vi "v0.2_vout_serial.vi"(8 "error in (no error)":errorcluster, 10 "Volt":dbl, 11 "VISA COM IN":refnum<visa-resource-name>) -> (0 "error out":errorcluster, 3 "VISA COM OUT":refnum<visa-resource-name>)   [LabVIEW 2011]
doc: "<B>Control de Velocidad</B>\n\nCabia el voltaje a la salida del amplificador operacional. Esto controla la velocidad del servomotor cuando se lo configura en modo de Control de Velocidad\n<B>Vout</B> Un valor entre -10 y 10 V"
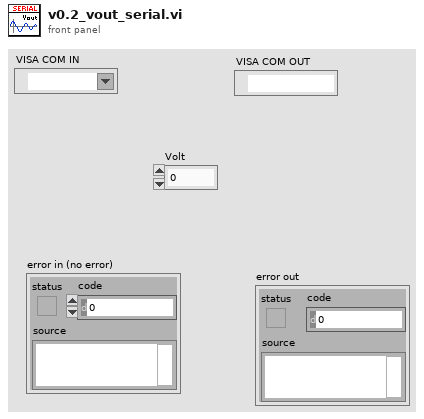
[diagram p1: front panel]
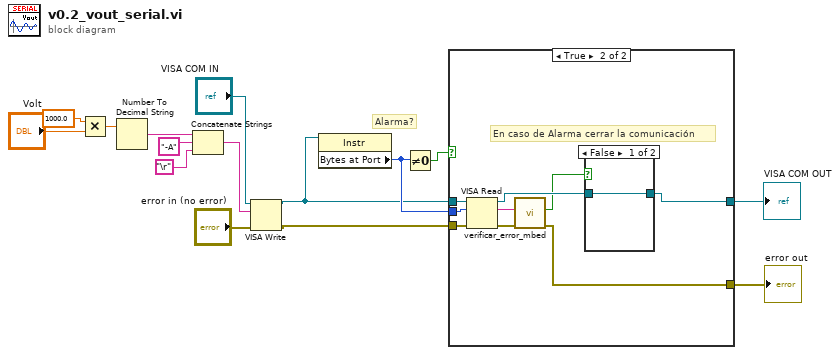
[diagram p0: block diagram]
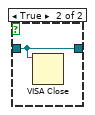
[diagram p3: hidden frame]
diagram:
  # "Alarma?"
  n1 = Multiply(x=1000.0, y="Volt") -> (x*y=w12:dbl)
  n2 = Number To Decimal String(number=w12) -> (decimal integer string=w11:string)  [unwired: 1 in]
  n3 = Concatenate Strings(w11, "-A" ("string"), "\r") -> (w9:string)
  n4 = VISA Write(VISA resource name="VISA COM IN", write buffer=w9, error in (no error)="error in (no error)") -> (VISA resource name out=w3:refnum<visa-resource-name>, error out=w4:errorcluster)  [unwired: 1 out]
  n5 = property class="Instr"(reference=w3) -> ("Bytes at Port"=w5:u32)  [unwired: 1 in, 2 out]
  n6 = Not Equal To 0?(x=w5) -> (x != 0?=w6:bool)
  n7 = case shown="True" w6 {
    tunnel: w3 -> [w17 w23]
    tunnel: w4 -> [w16 w22]
    tunnel: w5 -> [_ w20]
    tunnel: [w17 w19] -> w2
    tunnel: [w16 w18] -> w1
    frame False {
    }
    frame True {
      # "En caso de Alarma cerrar la comunicación"
      n8 = VISA Read(VISA resource name=w23, byte count=w20, error in (no error)=w22) -> (VISA resource name out=w24:refnum<visa-resource-name>, read buffer=w25:string, error out=w26:errorcluster)  [unwired: 1 out]
      n9 = call "verificar_error_mbed.vi"("error in (no error)"=w26, "desde_mbed"=w25) -> ("error out"=w18:errorcluster, "error?"=w21:bool)  [unwired: 8 in]
      n10 = case shown="False" w21 {
        tunnel: w24 -> [w27 w28]
        tunnel: [w27 w28] -> w19
        frame False {
        }
        frame True {
          n11 = VISA Close(VISA resource name=w28) -> ()  [unwired: 1 in, 1 out]
        }
      }
    }
  }
  "VISA COM OUT" <- w2
  "error out" <- w1
